vi "y_axisPID_ALB.vi"(7 "First Call?: T/F":bool, 10 "y axis":dbl) -> (2 "y axis out":dbl)   [LabVIEW 2017]
uses:
  <vilib>/addons/control/pid/NI_PID_pid.lvlib
  <vilib>/addons/control/pid/pid.llb/PID (DBL).vi
  <vilib>/addons/control/pid/pid.llb/PID Output Rate Limiter (DBL).vi
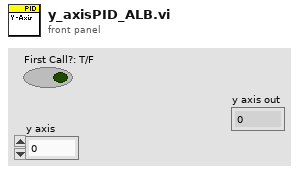
[diagram p1: front panel]
types:
  T1 = cluster{"P":dbl, "I":dbl, "derivative time (Td, min)":dbl}
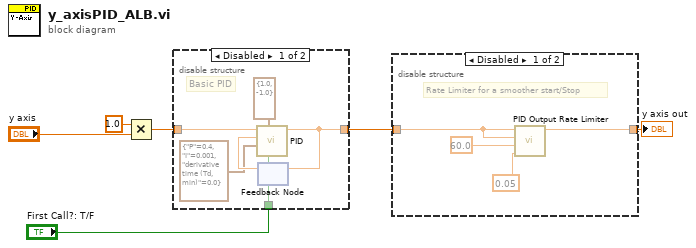
[diagram p0: block diagram]
diagram:
  n1 = Multiply(x=1.0, y="y axis") -> (x*y=w5:dbl)
  n2 = disable-structure shown="Disabled" {
    disable-tunnel: w5 -> [w12 w13]
    disable-tunnel: [w11 w13] -> w2
    disable-tunnel: "First Call?: T/F" -> [w7 _]
    frame Disabled {
      # "Basic PID"
      n3 = feedback #1() -> (w10:dbl)  [unwired: 1 in]
      n4 = call-poly <vilib>:"PID.vi"("reinitialize? (F)"=w7, "output range"=cluster{"output high":dbl, "output low":dbl} {"output high"=1.0, "output low"=-1.0}, "PID gains"=T1 {"P"=0.4, "I"=0.001, "derivative time (Td, min)"=0.0}, "process variable"=w10, "setpoint"=w12) -> ("output"=w11:dbl)  [unwired: 5 in, 1 out]
      n5 = feedback-in #1(w11) -> ()
    }
    frame Enabled {
    }
  }
  n6 = disable-structure shown="Disabled" {
    disable-tunnel: w2 -> [w16 w18]
    disable-tunnel: [w15 w18] -> w1
    frame Disabled {
      # "Rate Limiter for a smoother start/Stop"
      n7 = call-poly <vilib>:"PID Output Rate Limiter.vi"("dt (s)"=0.05, "output rate (EGU/min)"=60.0, "initial output"=w16, "input (controller output)"=w16) -> ("output"=w15:dbl)  [unwired: 4 in, 1 out]
    }
    frame Enabled {
    }
  }
  "y axis out" <- w1
